vi "AppendNewPackets.vi"(4 "PacketIDs":u32[](array[numeric]), 6 "SampleLen":i32, 7 "SamplesInPacketNrLen":i32, 8 "ErrorIn":errorcluster, 9 "PacketsNum":u32, 10 "PacketsIn":T1[](array[typedef]), 11 "FrameIn":string) -> (0 "ErrorOut":errorcluster, 2 "FrameOut":string, 3 "PacketsOut":T1[](array[typedef]))   [LabVIEW 2016]
doc: "Convert input frame (string) and append new packets to the packet array. \n\nIf error occurs or is at the input, the VI ends execution."
uses:
  FallSensor/Packet.ctl
  FallSensor/Sample.ctl
  FallSensor/Reading.ctl
  FallSensor/ReadingUnits/AccelReadingUnit.ctl
  FallSensor/ReadingUnits/GyroReadingUnit.ctl
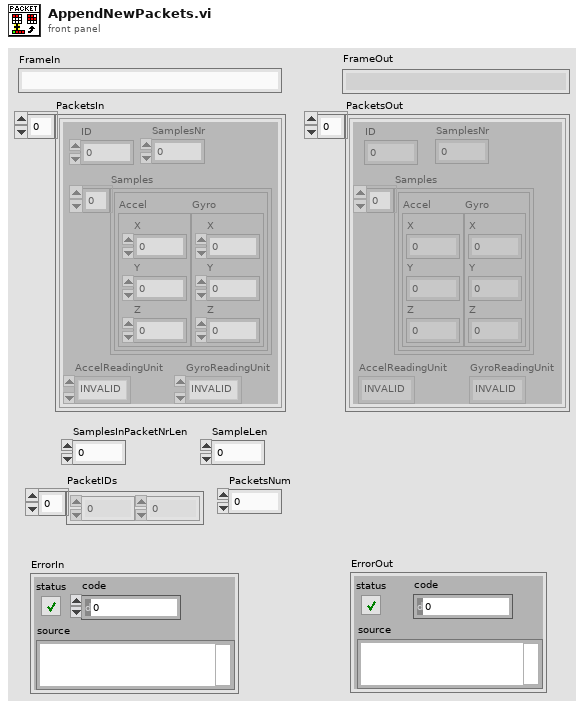
[diagram p1: front panel]
types:
  T1 = typedef "Packet.ctl" = cluster{"ID":u32, "SamplesNr":u32, "Samples":T2[], "AccelReadingUnit":T4, "GyroReadingUnit":T5}
  T2 = typedef "Sample.ctl" = cluster{"Accel":T3, "Gyro":T3}
  T3 = typedef "Reading.ctl" = cluster{"X":i16, "Y":i16, "Z":i16}
  T4 = typedef "AccelReadingUnit.ctl" = enum16{"INVALID", "RAW", "g"}
  T5 = typedef "GyroReadingUnit.ctl" = enum16{"INVALID", "RAW", "°/sec"}
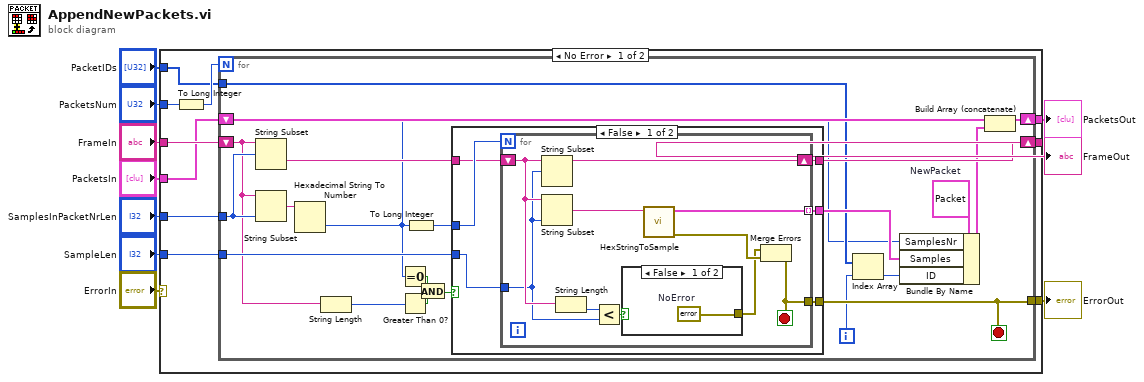
[diagram p0: block diagram]
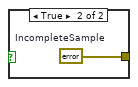
[diagram p2: hidden frame]
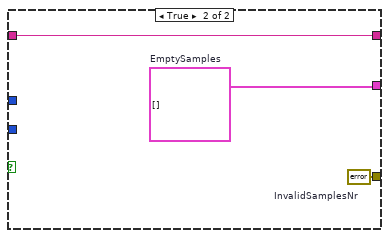
[diagram p3: hidden frame]
diagram:
  n1 = case shown="No Error" "ErrorIn" {
    selector: "ErrorIn" -> [_ w65]
    tunnel: "FrameIn" -> [w20 w64]
    tunnel: "PacketsNum" -> [w18 _]
    tunnel: [w14 w65] -> w7
    tunnel: "SamplesInPacketNrLen" -> [w17 _]
    tunnel: "SampleLen" -> [w16 _]
    tunnel: [w15 w64] -> w4
    tunnel: "PacketsIn" -> [w13 w63]
    tunnel: [w12 w63] -> w2
    tunnel: "PacketIDs" -> [w11 _]
    frame No Error {
      n2 = To Long Integer(number=w18) -> (32bit integer=w19:i32)
      n3 = for {
        N: w19 -> [_]
        shift-right: [w28] -> w12
        shift-left: w13 -> [w29]
        tunnel: w17 -> [w40]
        tunnel: w16 -> [w39]
        shift-right: [w37] -> w15
        shift-left: w20 -> [w34]
        tunnel: [w35] -> w14
        tunnel: w11 -> [w23]
        i -> [w22]
        stop <- w35 stop-if-true
        w27 = T1 {"ID"=0, "SamplesNr"=0, "Samples"=[], "AccelReadingUnit"=enum."INVALID", "GyroReadingUnit"=enum."INVALID"}  # NewPacket
        n4 = String Subset(string=w34, offset (0)=w40) -> (substring=w38:string)  [unwired: 1 in]
        n5 = String Subset(string=w34, length (rest)=w40) -> (substring=w41:string)  [unwired: 1 in]
        n6 = Hexadecimal String To Number ("HexStringToNumber")(string=w41) -> (number=w21:u32)  [unwired: 2 in, 1 out]
        n7 = String Length(string=w34) -> (length=w33:i32)
        n8 = Equal To 0?(x=w21) -> (x = 0?=w30:bool)
        n9 = Greater Than 0?(x=w33) -> (x > 0?=w31:bool)
        n10 = To Long Integer(number=w21) -> (32bit integer=w36:i32)
        n11 = And(x=w30, y=w31) -> (x .and. y?=w32:bool)
        n12 = case shown="False" w32 {
          tunnel: [w43 w62] -> w35
          tunnel: w39 -> [w45 _]
          tunnel: w38 -> [w46 w61]
          tunnel: [w44 w61] -> w37
          tunnel: w36 -> [w47 _]
          tunnel: [w42 w60] -> w26
          frame False {
            n13 = for {
              N: w47 -> [_]
              tunnel: w45 -> [w53]
              shift-right: [w57] -> w44
              shift-left: w46 -> [w55]
              tunnel: [w51] -> w43
              tunnel: [w48] -> w42 mode=indexing
              stop <- w51 stop-if-true
              n14 = String Subset(string=w55, offset (0)=w53) -> (substring=w57:string)  [unwired: 1 in]
              n15 = String Subset(string=w55, length (rest)=w53) -> (substring=w56:string)  [unwired: 1 in]
              n16 = String Length(string=w55) -> (length=w54:i32)
              n17 = Less?(x=w54, y=w53) -> (x < y?=w52:bool)
              n18 = case shown="False" w52 {
                tunnel: [w58 w59] -> w49
                frame False {
                  w58 = errorcluster {"status"=FALSE, "code"=0, "source"=""}  # NoError
                }
                frame True {
                  w59 = errorcluster {"status"=TRUE, "code"=5, "source"="Incomplete sample"}  # IncompleteSample
                }
              }
              n19 = call "HexStringToSample.vi"("StringIn"=w56) -> ("ErrorOut"=w50:errorcluster, "Sample"=w48:T2)  [unwired: 8 in, 1 out]
              n20 = Merge Errors(w49, w50) -> (w51:errorcluster)
            }
          }
          frame True {
            w60 = T2[] []  # EmptySamples
            w62 = errorcluster {"status"=TRUE, "code"=3, "source"="Invalid samples number"}  # InvalidSamplesNr
          }
        }
        n21 = Index Array(array=w23, index=w22) -> (element=w24:u32)
        n22 = Bundle By Name(cluster=w27, "SamplesNr"=w21, "Samples"=w26, "ID"=w24) -> (w25:T1)
        n23 = Build Array (concatenate)(w29, w25) -> (w28:T1[])
      }
    }
    frame Error {
    }
  }
  "PacketsOut" <- w2
  "ErrorOut" <- w7
  "FrameOut" <- w4
